vi "HPRF Signal Rescaler.vi"(4 "Signals":dbl[][](array[numeric])) -> (1 "Rescaled Signals":dbl[][](array[numeric]))   [LabVIEW 2013]
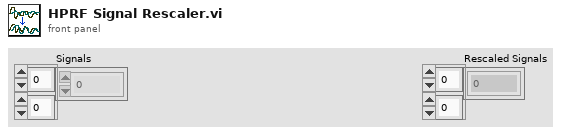
[diagram p1: front panel]
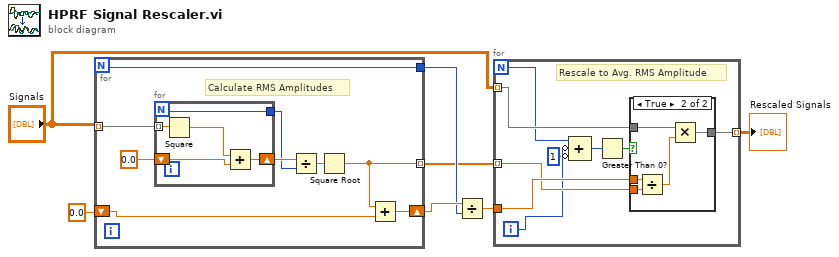
[diagram p0: block diagram]
diagram:
  n1 = for {
    N -> [w16]
    tunnel: "Signals" -> [w15] mode=indexing
    shift-right: [w10] -> w6
    shift-left: 0.0 ("element") -> [w8]
    tunnel: [w16] -> w5
    tunnel: [w9] -> w4 mode=indexing
    # "Calculate RMS Amplitudes"
    n2 = for {
      N -> [w17]
      tunnel: w15 -> [w21] mode=indexing
      shift-right: [w20] -> w13
      shift-left: 0.0 ("element") -> [w18]
      tunnel: [w17] -> w12
      n3 = Square(x=w21) -> (x^2=w19:dbl)
      n4 = Add(x=w19, y=w18) -> (x+y=w20:dbl)
    }
    n5 = Divide(x=w13, y=w12) -> (x/y=w11:dbl)
    n6 = Square Root(x=w11) -> (sqrt(x)=w9:dbl)
    n7 = Add(x=w9, y=w8) -> (x+y=w10:dbl)
  }
  n8 = Divide(x=w6, y=w5) -> (x/y=w3:dbl)
  n9 = for {
    N -> [w26]
    tunnel: w4 -> [w29] mode=indexing
    tunnel: "Signals" -> [w28] mode=indexing
    tunnel: w3 -> [w30]
    tunnel: [w27] -> w1 mode=indexing
    i -> [w25]
    # "Rescale to Avg. RMS Amplitude"
    n10 = Compound Arithmetic op=ADD(w26, invert w25, invert 1 ("value")) -> (w22:i32)
    n11 = Greater Than 0?(x=w22) -> (x > 0?=w23:bool)
    n12 = case shown="True" w23 {
      tunnel: w30 -> [_ w36]
      tunnel: w29 -> [_ w35]
      tunnel: w28 -> [w31 w34]
      tunnel: [w31 w32] -> w27
      frame False {
      }
      frame True {
        n13 = Divide(x=w36, y=w35) -> (x/y=w33:dbl)
        n14 = Multiply(x=w34, y=w33) -> (x*y=w32:dbl[])
      }
    }
  }
  "Rescaled Signals" <- w1
